vi "USRP_RXInit.vi"(0 "device names":refnum<k15>, 1 "USRP ControledParameters":T1={"active antenna"="TX1", "gain"=0.0, "carrier frequency"=100000.0, "IQ rate"=100000.0, "Active channels"="0,1"} {"IQ rate" format="%#_6p"; "carrier frequency" format="%#_6p"; "gain" format="%#_6f"}, 3 "error in (no error)":errorcluster) -> (7 "session handle out":refnum<k15>, 8 "USRP CoercedParamters":T2={"coerced IQ rate"=100000.0, "coerced carrier frequency"=100000.0, "coerced gain"=0.0} {"coerced gain" format="%#_6f"; "coerced carrier frequency" format="%#_6p"; "coerced IQ rate" format="%#_6p"}, 10 "error out":errorcluster)   [LabVIEW 2022 SP3]
panel:
  out "gain":dbl
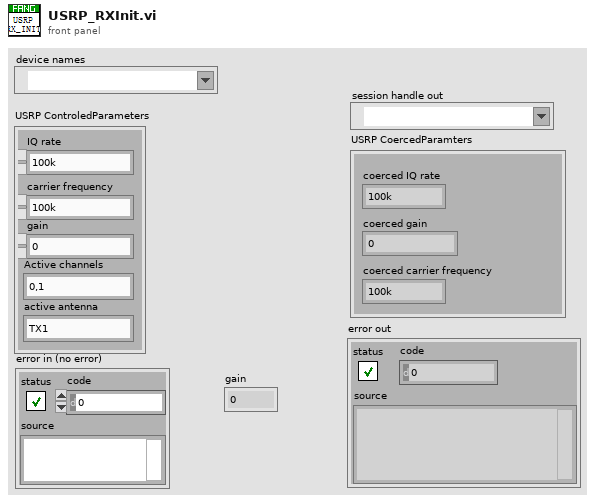
[diagram p1: front panel]
types:
  T1 = cluster{"active antenna":string, "gain":dbl, "carrier frequency":dbl, "IQ rate":dbl, "Active channels":string}
  T2 = cluster{"coerced IQ rate":dbl, "coerced carrier frequency":dbl, "coerced gain":dbl}
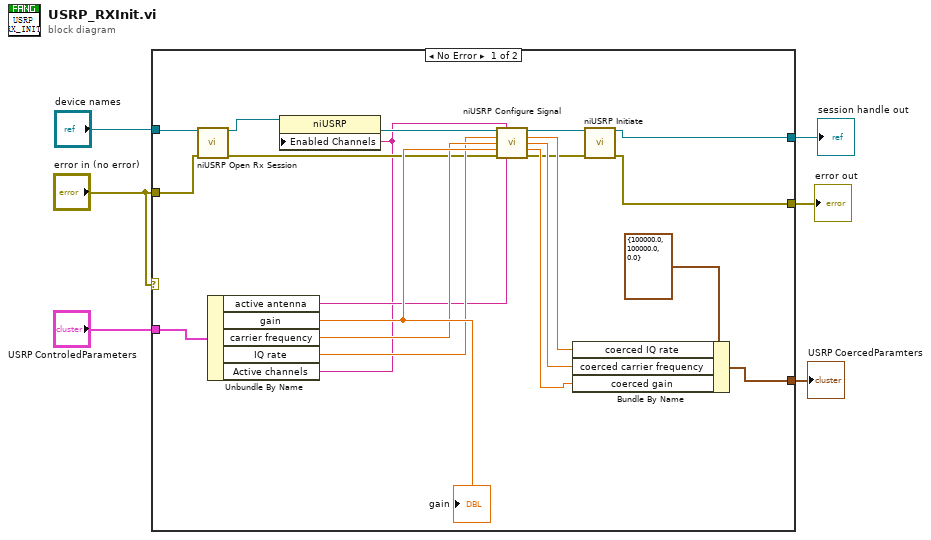
[diagram p0: block diagram]
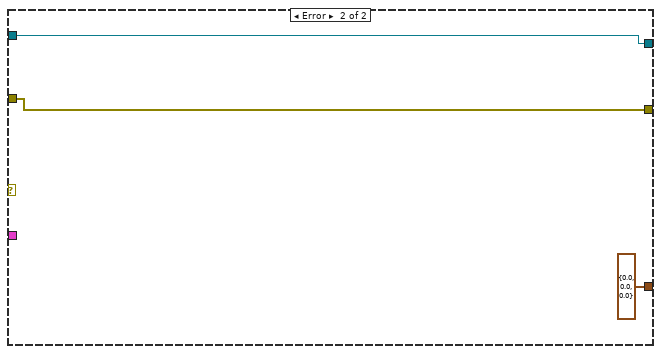
[diagram p2: hidden frame]
diagram:
  n1 = case shown="No Error" "error in (no error)" {
    tunnel: [w23 T2 {"coerced IQ rate"=0.0, "coerced carrier frequency"=0.0, "coerced gain"=0.0} ("USRP CoercedParamters")] -> w6
    tunnel: "USRP ControledParameters" -> [w18 _]
    tunnel: "device names" -> [w17 w28]
    tunnel: "error in (no error)" -> [w16 w29]
    tunnel: [w13 w29] -> w3
    tunnel: [w12 w28] -> w2
    frame No Error {
      n2 = call <instrlib>:"niUSRP Open Rx Session.vi"("device names"=w17, "error in (no error)"=w16) -> ("session handle out"=w9:refnum<k15>, "error out"=w15:errorcluster)  [unwired: 12 in]
      n3 = Unbundle By Name(w18) -> ("active antenna"=w10:string, "gain"=w26:dbl, "carrier frequency"=w25:dbl, "IQ rate"=w24:dbl, "Active channels"=w7:string)
      "gain" <- w26
      n4 = property class="niUSRP"(reference=w9, "Enabled Channels"=w7) -> (reference out=w8:refnum<k15>)  [unwired: 1 in, 1 out]
      n5 = call <instrlib>:"niUSRP Configure Signal.vi"("session handle"=w8, "channel list"=w7, "IQ rate"=w24, "carrier frequency"=w25, "gain"=w26, "error in (no error)"=w15, "active antenna"=w10) -> ("session handle out"=w11:refnum<k15>, "coerced IQ rate"=w22:dbl, "coerced carrier frequency"=w21:dbl, "coerced gain"=w20:dbl, "error out"=w14:errorcluster)  [unwired: 4 in]
      n6 = Bundle By Name(cluster=T2 {"coerced IQ rate"=100000.0, "coerced carrier frequency"=100000.0, "coerced gain"=0.0} ("USRP CoercedParamters"), "coerced IQ rate"=w22, "coerced carrier frequency"=w21, "coerced gain"=w20) -> (w23:T2)
      n7 = call <instrlib>:"niUSRP Initiate.vi"("session handle"=w11, "error in (no error)"=w14) -> ("session handle out"=w12:refnum<k15>, "error out"=w13:errorcluster)  [unwired: 12 in]
    }
    frame Error {
    }
  }
  "session handle out" <- w2
  "error out" <- w3
  "USRP CoercedParamters" <- w6
